vi "Pre Loop Init.vi"(8 "error in":errorcluster, 10 "Ref In":refnum<vi>) -> (0 "error out":errorcluster, 3 "Event Registration Refnum":refnum<event-registration>)   [LabVIEW 2018, in "Controller.lvlib"]
uses:
  Controller.lvlib
  Private Controls/Module Data Cluster.ctl
  Private Controls/Module Action.ctl
  User Events/controls/Actions.ctl
  Private Controls/Queue FG Action.ctl
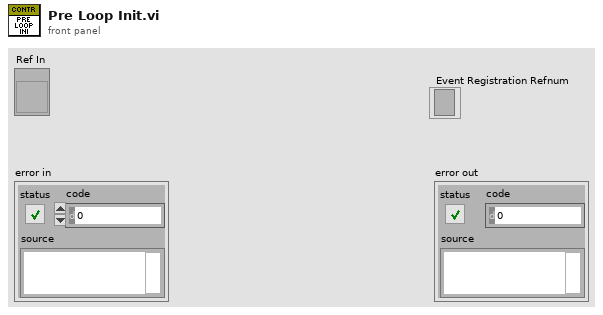
[diagram p1: front panel]
types:
  T1 = typedef "Controller.lvlib/Queue FG Action.ctl" = enum16{"Release", "Get", "Set"}
  T2 = typedef "Actions.ctl" = enum16{"Get", "Create", "Destroy"}
  T3 = typedef "Controller.lvlib/Module Data Cluster.ctl" = cluster{"Variant":variant, "action":T4}
  T4 = typedef "Controller.lvlib/Module Action.ctl" = enum16{"error", "exit", "init", "start", "Action", "Receive Config Data"}
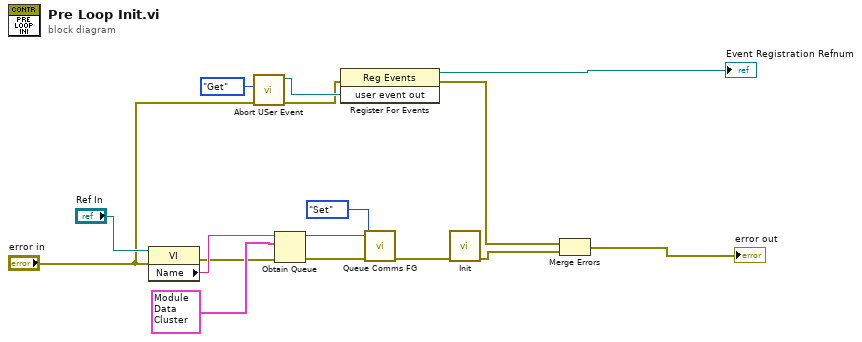
[diagram p0: block diagram]
diagram:
  n1 = property class="VI"(reference="Ref In", error in="error in") -> (error out=w9:errorcluster, "Name"=w15:string)  [unwired: 1 out]
  n2 = call "Abort USer Event.vi"("error in"="error in", "Enum"=Actions."Get") -> ("error out"=w3:errorcluster, "user event out"=w6:refnum<user-event>)  [unwired: 8 in]
  n3 = Obtain Queue(name (unnamed)=w15, element data type=T3 {"Variant"=variant, "action"=enum."init"} ("Module Data Cluster"), error in (no error)=w9) -> (queue out=w1:refnum<queue>, error out=w13:errorcluster)  [unwired: 2 in, 1 out]
  n4 = register-events(error in=w3, w6) -> (reference out=→"Event Registration Refnum":refnum<event-registration>, error out=w5:errorcluster)  [unwired: 1 in]
  n5 = call "Queue Comms FG.vi"("error in"=w13, "Action"=Queue_FG_Action."Set", "queue in"=w1) -> ("error out"=w12:errorcluster)  [unwired: 7 in, 1 out]
  n6 = call "Init.vi"("error in"=w12) -> ("error out"=w11:errorcluster)  [unwired: 10 in]
  n7 = Merge Errors(w5, w11) -> (→"error out":errorcluster)
